vi "geometry_controller.vi"(2 "Omga_prev":dbl[](array[numeric]), 3 "W":dbl[](array[numeric]), 4 "Cluster":cluster{"Y_sys":dbl[][], "eR":dbl[], "eW":dbl[]}, 5 "theta_hat":dbl[](array[numeric])) -> (0 "Omega_now":dbl[](array[numeric]), 1 "M":dbl[](array[numeric]))   [LabVIEW 2018]
uses:
  <vilib>/imath/engines/lvmath2/RunTimeEngine/BuiltInFunctions/diag/NIMS_diag.vi
  <instcachedir>/0/NIMS_diag_A176D428AACC4FD18ED77B06CA0A1FE1.lvgen/NIMS_diag_A176D428AACC4FD18ED77B06CA0A1FE1_003.vi
  <vilib>/imath/engines/lvmath2/RunTimeEngine/BuiltInFunctions/inv/NIMS_inv(GM).vi
  <instcachedir>/0/NIMS_inv(GM)_A6DF8FE880224208AACFE4CF9F659502.lvgen/NIMS_inv(GM)_A6DF8FE880224208AACFE4CF9F659502_000.vi
  <vilib>/imath/engines/lvmath2/RunTimeEngine/ErrorHandling/NIMS_Error From Error Code.vi
  <vilib>/imath/engines/lvmath2/RunTimeEngine/BuiltInFunctions/reshapemx/NIMS_[GV]_reshapemx.vi
  <instcachedir>/0/NIMS_[GV]_reshapemx_FC3E9BFA29934BE8A99DD7B75AE8F89C.lvgen/NIMS_[GV]_reshapemx_FC3E9BFA29934BE8A99DD7B75AE8F89C_000.vi
  <vilib>/imathl/engines/lvmath/Functions/Error Handling/Create Error.vi
  <vilib>/imath/engines/lvmath2/RunTimeEngine/IndexRead/NIMS V(S).vi
  <instcachedir>/0/NIMS V(S)_0488751826AF41519A22953C041130DC.lvgen/NIMS V(S)_0488751826AF41519A22953C041130DC_000.vi
  <vilib>/imath/engines/lvmath2/RunTimeEngine/ErrorHandling/NIMS_Create Error From Enums.vi
  <vilib>/imath/engines/lvmath2/RunTimeEngine/ArithmeticOperatorToken/NIMS_ArithmeticOperator_multmx-internal.vi
  <instcachedir>/0/NIMS_ArithmeticOperator_multmx-internal_16A6E1DA326644AB974D30232E729C42.lvgen/NIMS_ArithmeticOperator_multmx-internal_16A6E1DA326644AB974D30232E729C42_004.vi
  <vilib>/imath/engines/lvmath2/RunTimeEngine/ArithmeticOperatorToken/NIMS_ArithmeticOperator_multmx(M,CV).vi
  <instcachedir>/0/NIMS_ArithmeticOperator_multmx(M,CV)_2F1CD6A2FE4F4213A4AD1C901C2750F5.lvgen/NIMS_ArithmeticOperator_multmx(M,CV)_2F1CD6A2FE4F4213A4AD1C901C2750F5_000.vi
  <instcachedir>/0/NIMS_ArithmeticOperator_multmx(M,CV)_2F1CD6A2FE4F4213A4AD1C901C2750F5.lvgen/NIMS_ArithmeticOperator_multmx(M,CV)_2F1CD6A2FE4F4213A4AD1C901C2750F5_001.vi
  <vilib>/imath/engines/lvmath2/RunTimeEngine/ArithmeticOperatorToken/NIMS_ArithmeticOperator_minus.vi
  <instcachedir>/0/NIMS_ArithmeticOperator_minus_C4D0373119CC411691B2E50DF2E09F22.lvgen/NIMS_ArithmeticOperator_minus_C4D0373119CC411691B2E50DF2E09F22_002.vi
  <vilib>/imath/engines/lvmath2/RunTimeEngine/ArithmeticOperatorToken/NIMS_ArithmeticOperator_plus.vi
  <instcachedir>/0/NIMS_ArithmeticOperator_plus_DE670E32103C4C10ADF2A97367172B30.lvgen/NIMS_ArithmeticOperator_plus_DE670E32103C4C10ADF2A97367172B30_003.vi
  <vilib>/imath/engines/lvmath2/RunTimeEngine/MatrixToken/NIMS_MatrixToken_M_SorCV.vi
  <instcachedir>/0/NIMS_MatrixToken_M_SorCV_91F8B6182BA1450B95B3875CCE45F523.lvgen/NIMS_MatrixToken_M_SorCV_91F8B6182BA1450B95B3875CCE45F523_001.vi
  <vilib>/imath/engines/lvmath2/RunTimeEngine/RangeToken/NIMS_Range_R2 - Integer.vi
  <instcachedir>/0/NIMS_Range_R2 - Integer_E35B921DECF84AADB7325A02D418BFCC.lvgen/NIMS_Range_R2 - Integer_E35B921DECF84AADB7325A02D418BFCC_000.vi
  <vilib>/imath/engines/lvmath2/RunTimeEngine/CommandStatement/MC_CommandStatement_break.vi
  <vilib>/imath/engines/lvmath2/RunTimeEngine/IndexRead/NIMS M(S).vi
  <instcachedir>/0/NIMS M(S)_B826C018497E4940AE96BD27B540B6FB.lvgen/NIMS M(S)_B826C018497E4940AE96BD27B540B6FB_000.vi
  <vilib>/imath/engines/lvmath2/RunTimeEngine/IndexReplace/NIMS M(S)=S.vi
  <instcachedir>/0/NIMS M(S)=S_3A43114EBE4B4893BC108DAA709F76B8.lvgen/NIMS M(S)=S_3A43114EBE4B4893BC108DAA709F76B8_001.vi
  <vilib>/imath/engines/lvmath2/RunTimeEngine/ArithmeticOperatorToken/NIMS_ArithmeticOperator_multmx.vi
  <instcachedir>/0/NIMS_ArithmeticOperator_multmx_622CA76F9646436AB036D42A9A1CE0E6.lvgen/NIMS_ArithmeticOperator_multmx_622CA76F9646436AB036D42A9A1CE0E6_004.vi
  <vilib>/imath/engines/lvmath2/RunTimeEngine/NodeEndStatement/NIMS_NodeEndStatement_Get Vector.vi
  <instcachedir>/0/NIMS_NodeEndStatement_Get Vector_329D0992E87F49F089135171B7FC9327.lvgen/NIMS_NodeEndStatement_Get Vector_329D0992E87F49F089135171B7FC9327_001.vi
  <vilib>/imath/engines/lvmath/Functions/Error Handling/MergeErrorsWrapper.vi
  <vilib>/imath/engines/lvmath2/RunTimeEngine/NodeEndStatement/NIMS_NodeEndStatement_Output.vi
  <instcachedir>/0/NIMS_NodeEndStatement_Output_53EC0D466D134D7ABD903AC30B43404B.lvgen/NIMS_NodeEndStatement_Output_53EC0D466D134D7ABD903AC30B43404B_005.vi
  <vilib>/imath/engines/lvmath2/RunTimeEngine/ErrorHandling/NIMS_Finalize Error.vi
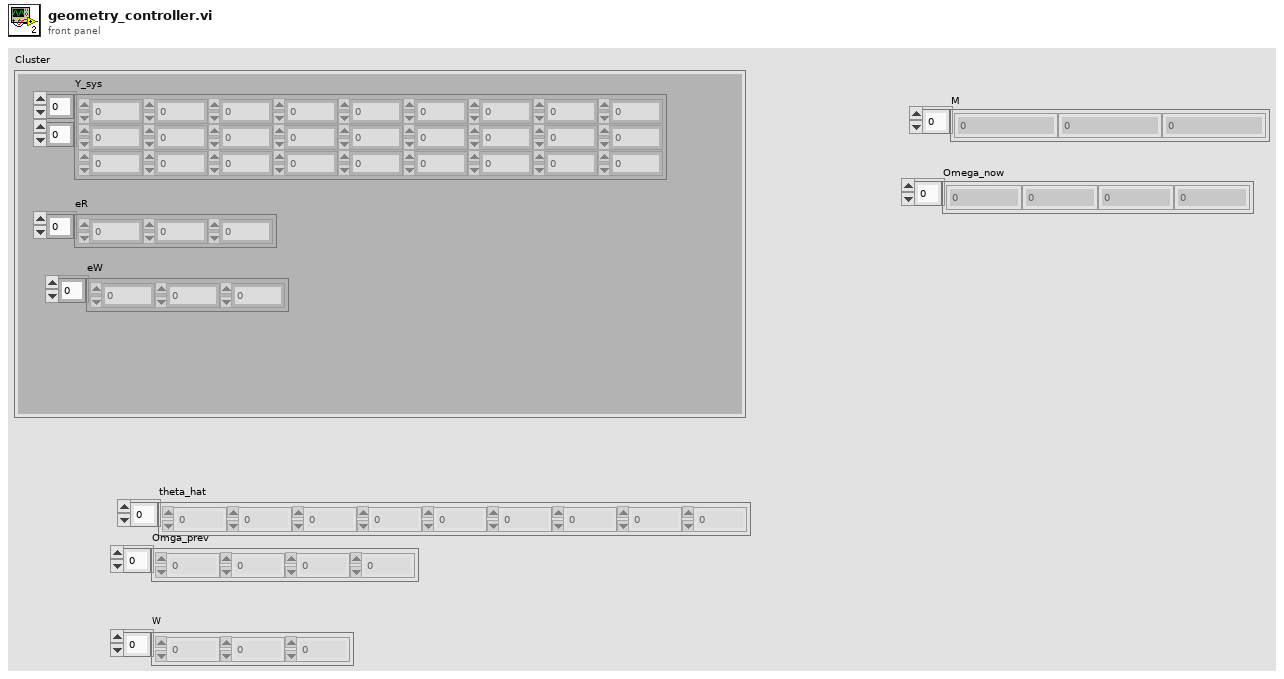
[diagram p1: front panel]
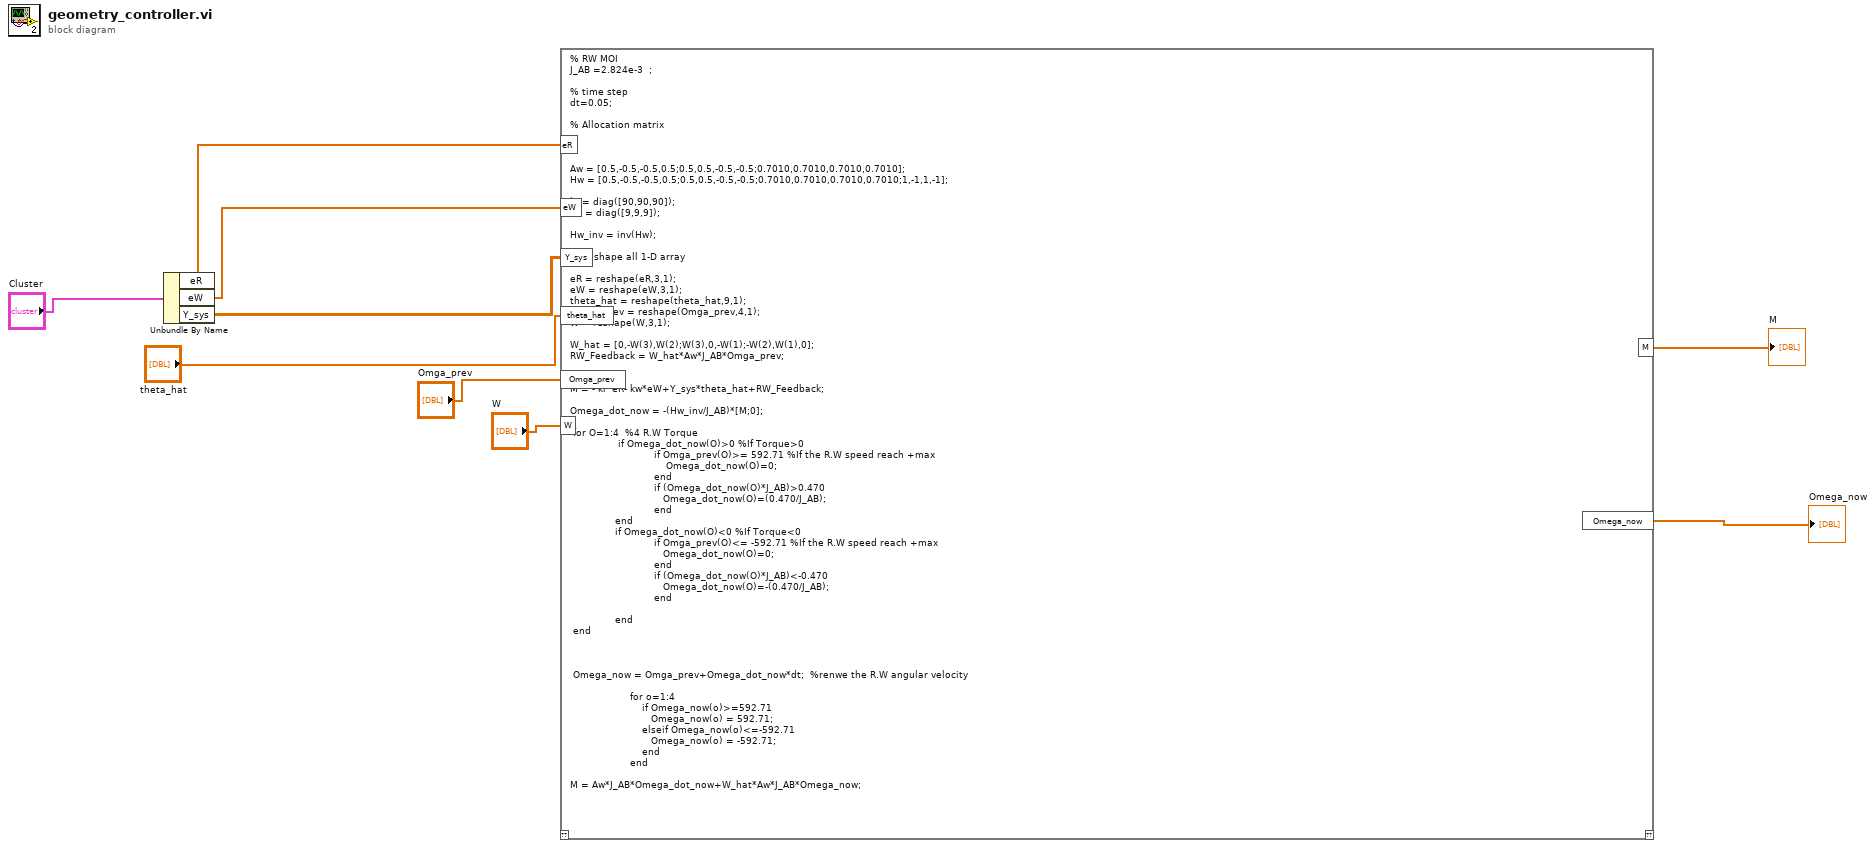
[diagram p0: block diagram]
diagram:
  n1 = Unbundle By Name("Cluster") -> ("eR"=w2:dbl[], "eW"=w3:dbl[], "Y_sys"=w4:dbl[][])
  n2 = mathscript code="% RW MOI\nJ_AB =2.824e-3  ;\n\n% time step\ndt=0.05;\n\n% Allocation matrix\n\n\n\nAw = [0.5,-0.5,-0.5,0.5;0.5,0.5,-0.5,-0.5;0.7010,0.7010,0.7010,0.7010];\nHw = [0.5,-0.5,-0.5,0.5;0.5,0.5,-0.5,-0.5;0.7010,0.7010,0.7010,0.7010;1,-1,1,-1];\n\nkr = diag([90,90,90]);\nkw = diag([9,9,9]);\n\nHw_inv = inv(Hw);\n\n% Reshape all 1-D array\n\neR = reshape(eR,3,1);\neW = reshape(eW,3,1);\ntheta_hat = reshape(theta_hat,9,1);\nOmga_prev = reshape(Omga_prev,4,1);\nW = reshape(W,3,1);\n\nW_hat = [0,-W(3),W(2);W(3),0,-W(1);-W(2),W(1),0];\nRW_Feedback = W_hat*Aw*J_AB*Omga_prev;\n\n\nM = - kr*eR- kw*eW+Y_sys*theta_hat+RW_Feedback;\n\nOmega_dot_now = -(Hw_inv/J_AB)*[M;0];\n\n for O=1:4  %4 R.W Torque\n                if Omega_dot_now(O)>0 %If Torque>0\n                            if Omga_prev(O)>= 592.71 %If the R.W speed reach +max\n                                Omega_dot_now(O)=0;\n                            end\n                            if (Omega_dot_now(O)*J_AB)>0.470\n                               Omega_dot_now(O)=(0.470/J_AB);\n                            end\n               end\n               if Omega_dot_now(O)<0 %If Torque<0\n                            if Omga_prev(O)<= -592.71 %If the R.W speed reach +max\n                               Omega_dot_now(O)=0;\n                            end\n                            if (Omega_dot_now(O)*J_AB)<-0.470\n                               Omega_dot_now(O)=-(0.470/J_AB);\n                            end\n\n               end\n end\n                  \n                    \n                   \n Omega_now = Omga_prev+Omega_dot_now*dt;  %renwe the R.W angular velocity\n                   \n                    for o=1:4\n                        if Omega_now(o)>=592.71\n                           Omega_now(o) = 592.71;\n                        elseif Omega_now(o)<=-592.71\n                           Omega_now(o) = -592.71; \n                        end\n                    end\n\nM = Aw*J_AB*Omega_dot_now+W_hat*Aw*J_AB*Omega_now;"("eR"=w2, "eW"=w3, "Y_sys"=w4, "theta_hat"="theta_hat", "Omga_prev"="Omga_prev", "W"="W") -> ("Omega_now"=→"Omega_now":dbl[], "M"=→"M":dbl[])  [unwired: 1 in, 1 out]
